vi "Get Keywords.vi"(8 "error in (no error)":errorcluster, 11 "UI Functions in":refnum<class "UI Functions.lvclass">) -> (0 "error out":errorcluster, 2 "Keywords":string[](array[string]), 3 "UI Functions out":refnum<class "UI Functions.lvclass">)   [LabVIEW 2019, in "UI Functions.lvclass"]
uses:
  UI Functions.lvclass
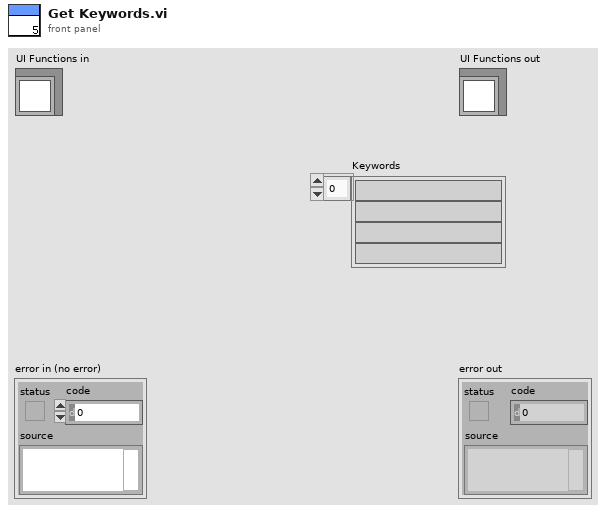
[diagram p1: front panel]
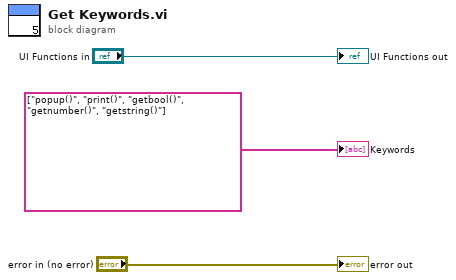
[diagram p0: block diagram]
diagram:
  "error out" <- "error in (no error)"
  "UI Functions out" <- "UI Functions in"
  "Keywords" <- string[] ["popup()", "print()", "getbool()", "getnumber()", "getstring()"] ("Keywords")
